vi "NXTLineLeader-Remote.vi"(10 "Base Power":i8=75 min=0 max=100, 12 "Base Direction":bool=TRUE) -> (15 "Motor 1 Power":u8, 16 "Boolean":bool caption="Yes / No", 17 "Motor 1 Direction":bool, 18 "Motor 2 Power":u8, 19 "Motor 2 Direction":bool)   [LabVIEW 2009]
uses:
  <vilib>/NXT/Block Support/NXT_InputPort.ctl
  <vilib>/NXT/Subs/LVHSConnector.ctl
  <vilib>/NXT/Subs/MotorOutput.ctl
  <vilib>/NXT/Block Support/NXT_OutputGoalType.ctl
  <vilib>/NXT/Block Support/NXT_OutputPort.ctl
panel:
  in  "Operation":u8(ring) items=["Track Line", "Read Raw Sensor ", "Read  Sensor Average "]
  out "NXT dup":T1={"error"={"status"=FALSE, "code"=0, "source"=""}, "address"="", "NXT #"=-1, "Show Error"=TRUE}
  in  "Utility Operation":u8(ring) caption="Operation" items=["Config PID Control", "Wakeup", "Sleep", "Take a Snapshot", "Invert Line to White", "Reset Inversion", "Calibrate White", "Calibrate Black"]
  in  "NXT":T1={"error"={"status"=FALSE, "code"=0, "source"=""}, "address"="", "NXT #"=-1, "Show Error"=TRUE}
  in  "Kd_factor":u8=32 min=1
  in  "Ki_factor":u8=32 min=1
  in  "Kp_factor":u8=32 min=1
  in  "SetPoint":u8=45 max=80
  in  "Kd":u8=15
  in  "Ki":u8
  in  "Kp":u8=25
  in  "Input Port":T2 items=["Port 1", "Port 2", "Port 3", "Port 4"]
  in  "MD2":string
  in  "MD1":string
  in  "Base Direction":string
  # "PID Control"
  # "mindsensors.com\nCopyright (c) 2009 by mindsensors.com\nEmail: info (<at>) mindsensors (<dot>) com\n\nThis program is free software. You can redistribute it and/or modify\nit under the terms of the GNU General Public License as published by\nthe Free Software Foundation; version 3 of the License.\nRead the license at: http://www.gnu.org/licenses/gpl.txt"
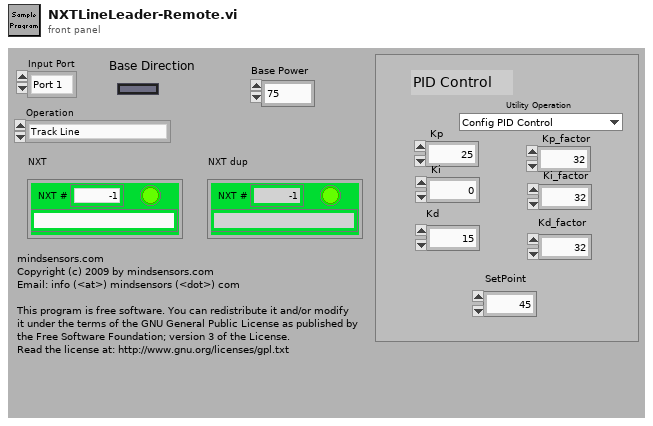
[diagram p1: front panel]
types:
  T1 = typedef "LVHSConnector.ctl" = cluster{"error":errorcluster, "address":string, "NXT #":i32, "Show Error":bool}
  T2 = typedef "NXT_InputPort.ctl" = u8
  T3 = typedef "NXT_OutputGoalType.ctl" = u16
  T4 = typedef "NXT_OutputPort.ctl" = u8
  T5 = typedef "MotorOutput.ctl" = u16
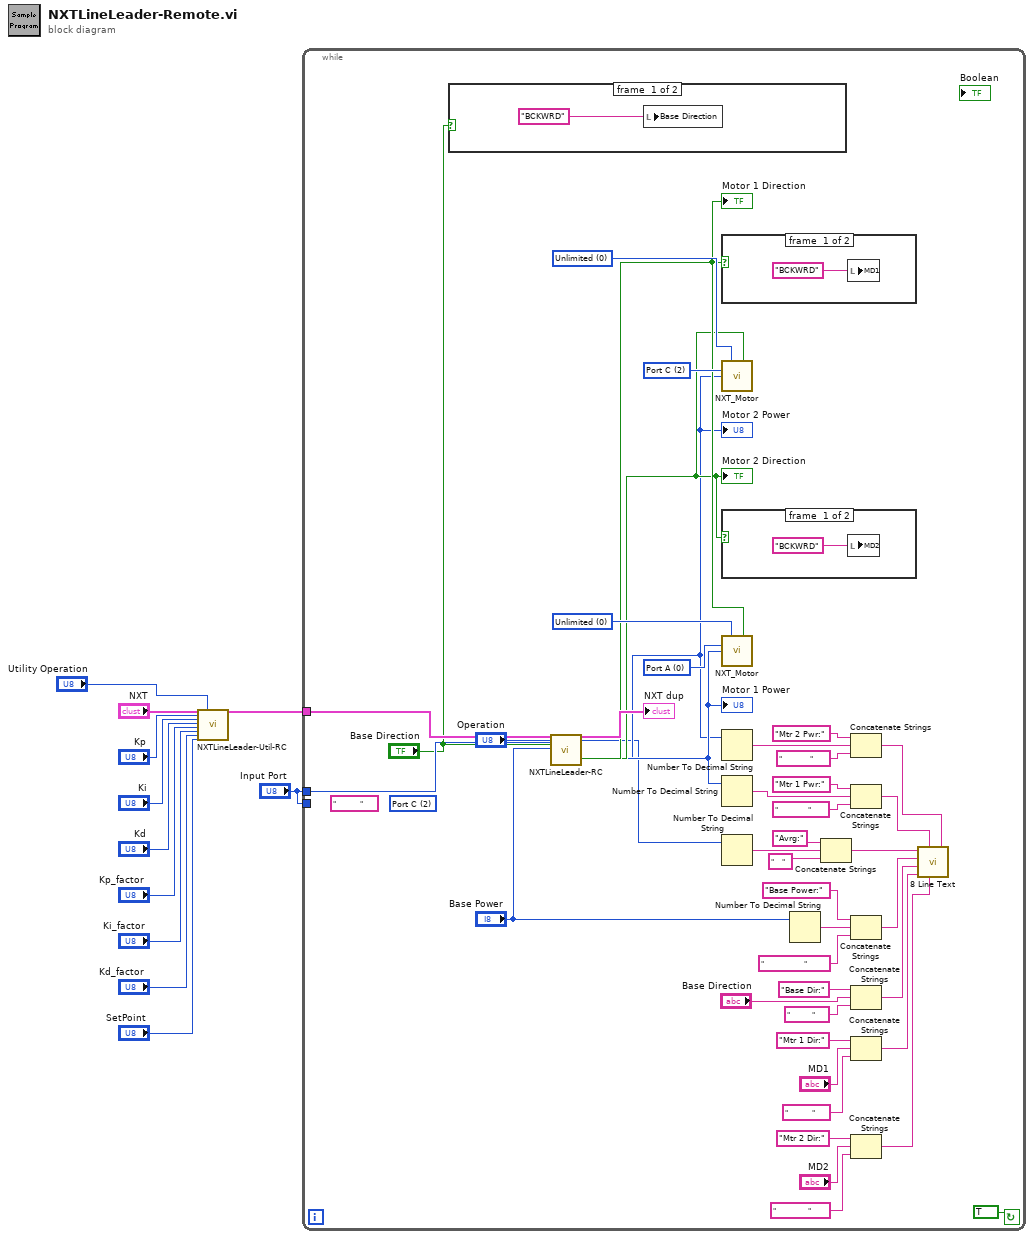
[diagram p0: block diagram]
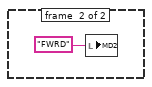
[diagram p2: hidden frame]
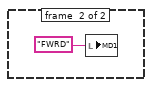
[diagram p3: hidden frame]
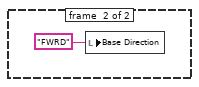
[diagram p4: hidden frame]
diagram:
  n1 = call "NXTLineLeader-Util-RC.vi"("NXT"="NXT", "Kp"="Kp", "Ki"="Ki", "Kd"="Kd", "Kp factor"="Kp_factor", "Ki factor"="Ki_factor", "Kd factor"="Kd_factor", "SetPoint"="SetPoint", "Operation"="Utility Operation") -> ("NXT dup"=w10:T1)  [unwired: 17 in, 1 out]
  n2 = while {
    tunnel: "Input Port" -> [_]
    tunnel: "Input Port" -> [w22]
    tunnel: w10 -> [w21]
    stop <- TRUE continue-if-true
    w27 = T3 0 items=["Unlimited", "Distance", "Time", "Stop"] ("Goal Type")
    w28 = T4 2 items=["Port A", "Port B", "Port C"] ("Output (Port A)")
    w29 = T4 0 items=["Port A", "Port B", "Port C"] ("Output (Port A)")
    w30 = T3 0 items=["Unlimited", "Distance", "Time", "Stop"] ("Goal Type")
    (unwired) T5 2 items=["Port A", "Port B", "Port C", "All Ports"] ("Output Port")
    (unwired) "            " ("string")
    n3 = case shown="False" "Base Direction" {
      frame #0 {
        n4 = local write "Base Direction"("BCKWRD") -> ()
      }
      frame #1 {
        n5 = local write "Base Direction"("FWRD") -> ()
      }
    }
    n6 = call "NXTLineLeader-RC.vi"("NXT"=w21, "Operation"="Operation", "Base Direction"="Base Direction", "Base Power"="Base Power", "Input Port"=w22) -> ("Motor 1 Direction"=w16:bool, "Motor 1 Power"=w14:u8, "Motor 2 Direction"=w15:bool, "Motor 2 Power"=w13:u8, "NXT dup"=→"NXT dup":T1, "Average Value"=w12:u8)  [unwired: 13 in, 4 out]
    "Motor 1 Power" <- w14
    "Motor 1 Direction" <- w16
    "Motor 2 Power" <- w13
    "Motor 2 Direction" <- w15
    n7 = case shown="False" w16 {
      frame #0 {
        n8 = local write "MD1"("BCKWRD") -> ()
      }
      frame #1 {
        n9 = local write "MD1"("FWRD") -> ()
      }
    }
    n10 = call "NXT_Motor.vi"("Goal Type"=w27, "Direction (T: Fwd)"=w15, "Output (Port A)"=w28, "Power"=w13) -> ()  [unwired: 8 in, 4 out]
    n11 = case shown="False" w15 {
      frame #0 {
        n12 = local write "MD2"("BCKWRD") -> ()
      }
      frame #1 {
        n13 = local write "MD2"("FWRD") -> ()
      }
    }
    n14 = call "NXT_Motor.vi"("Goal Type"=w30, "Direction (T: Fwd)"=w16, "Output (Port A)"=w29, "Power"=w14) -> ()  [unwired: 8 in, 4 out]
    n15 = Number To Decimal String(number=w13) -> (decimal integer string=w35:string)  [unwired: 1 in]
    n16 = Number To Decimal String(number=w14) -> (decimal integer string=w36:string)  [unwired: 1 in]
    n17 = Number To Decimal String(number=w12) -> (decimal integer string=w24:string)  [unwired: 1 in]
    n18 = Number To Decimal String(number="Base Power") -> (decimal integer string=w52:string)  [unwired: 1 in]
    n19 = Concatenate Strings("Avrg:" ("string"), w24, "    " ("string")) -> (w23:string)
    n20 = Concatenate Strings("Mtr 2 Pwr:" ("string"), w35, "              " ("string")) -> (w32:string)
    n21 = Concatenate Strings("Mtr 1 Pwr:" ("string"), w36, "               " ("string")) -> (w31:string)
    n22 = Concatenate Strings("Base Power:" ("string"), w52, "                    " ("string")) -> (w51:string)
    n23 = Concatenate Strings("Base Dir:" ("string"), "Base Direction", "           " ("string")) -> (w47:string)
    n24 = Concatenate Strings("Mtr 1 Dir:" ("string"), "MD1", "            " ("string")) -> (w40:string)
    n25 = Concatenate Strings("Mtr 2 Dir:" ("string"), "MD2", "                " ("string")) -> (w39:string)
    n26 = call "8 Line Text.vi"("Line 7"=w32, "Line 6"=w39, "Line 5"=w31, "Line 4"=w40, "Line 3"=w47, "Line 2"=w51, "Line 1"=w23) -> ()  [unwired: 1 in]
  }
